vi "Set_PScontrol_Cell.vi"(8 "error in (no error)":errorcluster, 10 "Command_Message_in":T2, 11 "Command_queue_in":T1) -> (0 "error out":errorcluster, 2 "Command_Message_out":T2, 3 "Command_queue_out":T1)   [LabVIEW 2019]
uses:
  Command_Message.ctl
  Command_Queue.ctl
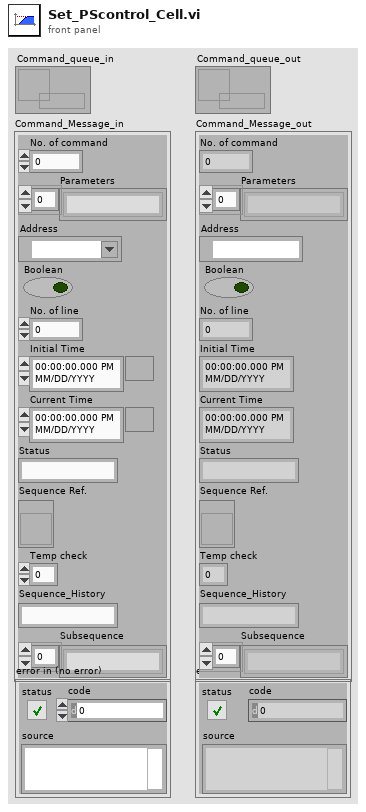
[diagram p1: front panel]
types:
  T1 = typedef "Command_Queue.ctl" = refnum<queue>
  T2 = typedef "Command_Message.ctl" = cluster{"No. of command":i32, "Parameters":string[], "Address":refnum<visa-resource-name>, "Boolean":bool, "No. of line":i32, "Initial Time":timestamp, "Current Time":timestamp, "Status":string, "Sequence Ref.":refnum<vi>, "Temp check":i32, "Sequence_History":string, "Subsequence":string[]}
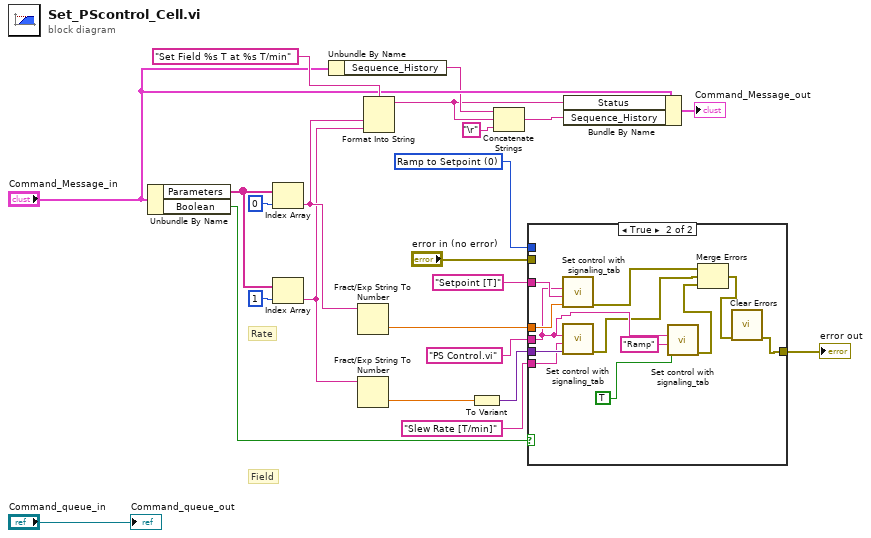
[diagram p0: block diagram]
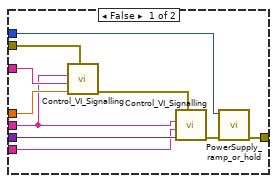
[diagram p2: hidden frame]
diagram:
  w17 = u16 0 items=["Ramp to Setpoint", "Hold"] ("Mode")
  # "Rate"
  # "Field"
  n1 = Unbundle By Name("Command_Message_in") -> ("Parameters"=w11:string[], "Boolean"=w4:bool)
  n2 = Index Array(array=w11, index=0) -> (element=w14:string)
  n3 = Index Array(array=w11, index=1) -> (element=w13:string)
  n4 = Unbundle By Name("Command_Message_in") -> ("Sequence_History"=w8:string)
  n5 = Fract/Exp String To Number(string=w14) -> (number=w21:dbl)  [unwired: 3 in, 1 out]
  n6 = Fract/Exp String To Number(string=w13) -> (number=w19:dbl)  [unwired: 3 in, 1 out]
  n7 = Format Into String(format string="Set Field %s T at %s T/min", w14, w13) -> (resulting string=w7:string)  [unwired: 2 in, 1 out]
  n8 = To Variant(anything=w19) -> (Variant=w18:variant)
  n9 = Concatenate Strings(w8, w7, "\r") -> (w5:string)
  n10 = case shown="True" w4 {
    tunnel: w21 -> [w27 w45]
    tunnel: "error in (no error)" -> [w33 _]
    tunnel: w18 -> [w31 w44]
    tunnel: w17 -> [w29 _]
    tunnel: [w28 w39] -> w16
    tunnel: "Setpoint [T]" -> [w26 w43]
    tunnel: "PS Control.vi" ("Target VI name") -> [w25 w41]
    tunnel: "Slew Rate [T/min]" ("Control Name") -> [w24 w42]
    frame False {
      n11 = call "Control_VI_Signalling.vi"("error in (no error)"=w33, "Input Value"=w27, "Control Name"=w26, "Target VI name"=w25) -> ("error out"=w32:errorcluster)  [unwired: 7 in]
      n12 = call "Control_VI_Signalling.vi"("error in (no error)"=w32, "Input Value"=w31, "Control Name"=w24, "Target VI name"=w25) -> ("error out"=w30:errorcluster)  [unwired: 7 in]
      n13 = call "PowerSupply_ramp_or_hold.vi"("error in (no error)"=w30, "Mode"=w29) -> ("error out"=w28:errorcluster)  [unwired: 9 in]
    }
    frame True {
      n14 = call "Set control with signaling_tab.vi"("Value (Signaling)"=w45, "Control Name"=w43, "VI Name"=w41) -> ("error out"=w37:errorcluster)  [unwired: 8 in]
      n15 = call "Set control with signaling_tab.vi"("Value (Signaling)"=w44, "Control Name"=w42, "VI Name"=w41) -> ("error out"=w36:errorcluster)  [unwired: 8 in]
      n16 = call "Set control with signaling_tab.vi"("Value (Signaling)"=TRUE, "Control Name"="Ramp", "VI Name"=w41) -> ("error out"=w35:errorcluster)  [unwired: 8 in]
      n17 = Merge Errors(w37, w36, w35) -> (w34:errorcluster)
      n18 = call <vilib>:"Clear Errors.vi"("error in (no error)"=w34) -> ("error out"=w39:errorcluster)  [unwired: 5 in, 1 out]
    }
  }
  "error out" <- w16
  n19 = Bundle By Name(cluster="Command_Message_in", "Status"=w7, "Sequence_History"=w5) -> (→"Command_Message_out":T2)
  "Command_queue_out" <- "Command_queue_in"
